vi "ke37xx Pattern Catalog.vi"(0 "VISA Resource Name":refnum<visa-resource-name>, 11 "error in (no error)":errorcluster, 12 "Bytes To Read (1024)":u32=1024) -> (4 "VISA Resource Name Out":refnum<visa-resource-name>, 8 "Patterns":string, 15 "error out":errorcluster)   [LabVIEW 2009, in "Keithley 3700 Series.lvlib"]
doc: "This VI allows you query the currently defined channel patterns."
uses:
  <instrlib>/Keithley 3706/Keithley 3700 Series.lvlib
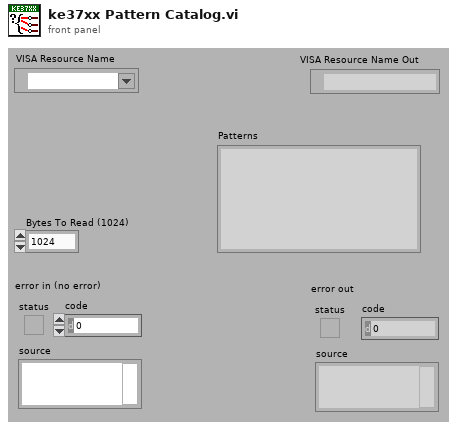
[diagram p1: front panel]
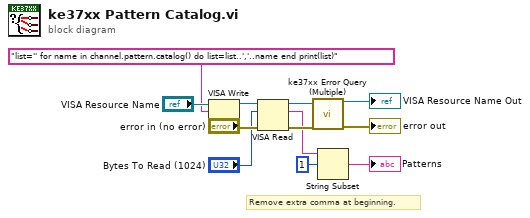
[diagram p0: block diagram]
diagram:
  # "Remove extra comma at beginning."
  n1 = VISA Write(VISA resource name="VISA Resource Name", write buffer="list='' for name in channel.pattern.catalog() do list=list..','..name end print(list)", error in (no error)="error in (no error)") -> (VISA resource name out=w6:refnum<visa-resource-name>, error out=w13:errorcluster)  [unwired: 1 out]
  n2 = VISA Read(VISA resource name=w6, byte count="Bytes To Read (1024)", error in (no error)=w13) -> (VISA resource name out=w5:refnum<visa-resource-name>, read buffer=w3:string, error out=w12:errorcluster)  [unwired: 1 out]
  n3 = call <instrlib>:"ke37xx Error Query (Multiple).vi"("VISA resource name"=w5, "error in (no error)"=w12) -> ("VISA resource name out"=→"VISA Resource Name Out":refnum<visa-resource-name>, "error out"=→"error out":errorcluster)  [unwired: 12 out]
  n4 = String Subset(string=w3, offset (0)=1) -> (substring=→"Patterns":string)  [unwired: 1 out]
